vi "Configure Frequency Voltage Range.vi"(6 "Display (0: Primary Display)":i32(ring) items=["Primary Display", "Secondary Display"], 8 "error in (no error)":errorcluster, 9 "Manual Range (10)":dbl=10.0, 10 "Enable Frequency Voltage Auto Range (T:Enable)":bool=TRUE, 11 "VISA resource name":refnum<visa-resource-name>) -> (0 "error out":errorcluster, 3 "VISA resource name out":refnum<visa-resource-name>)   [LabVIEW 2020, in "Agilent 34405.lvlib"]
doc: "Configures the voltage range for Frequency measurement on the instrument.\n\n<B>Notes:</B>\n(1) This VI is only valid if the measurement function is set to Frequency."
uses:
  <instrlib>/Agilent 34405/Agilent 34405.lvlib
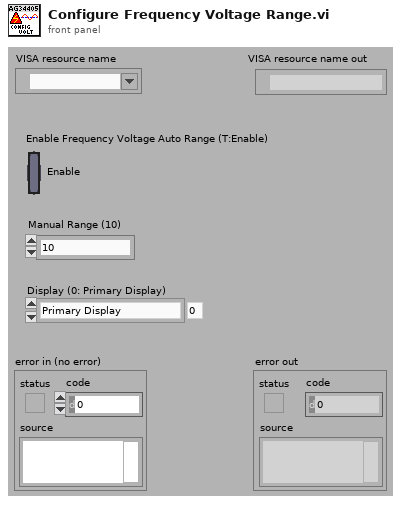
[diagram p1: front panel]
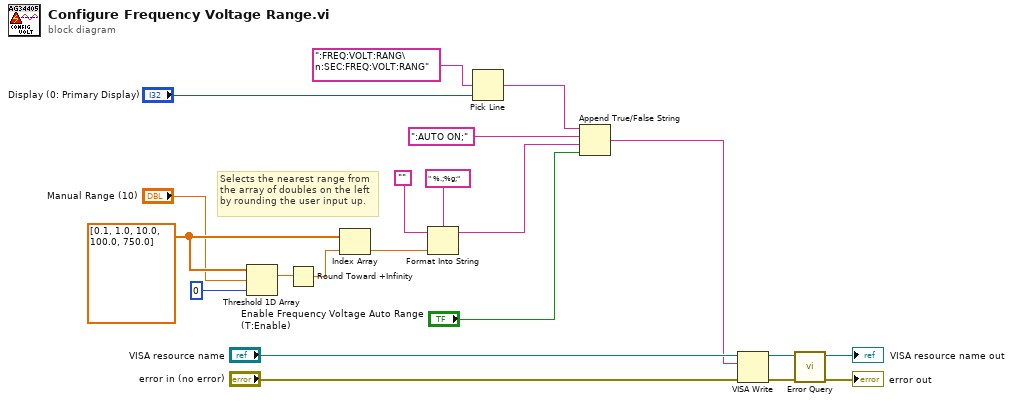
[diagram p0: block diagram]
diagram:
  w13 = dbl[] [0.1, 1.0, 10.0, 100.0, 750.0]
  # "Selects the nearest range from the array of doubles on the left by rounding the user input up."
  n1 = Threshold 1D Array(1:0 ("start index (0)"), 2:"Manual Range (10)", 3:w13) -> (0:w14:dbl)
  n2 = Round Toward +Infinity ("Round To +Infinity")(x=w14) -> (ceil(x): smallest int >= x=w12:dbl)
  n3 = Index Array(array=w13, index=w12) -> (element=w11:dbl)
  n4 = Format Into String(format string=" %.;%g;", initial string="" ("Empty String Constant"), w11) -> (resulting string=w6:string)  [unwired: 1 in, 1 out]
  n5 = Pick Line(multi-line string=":FREQ:VOLT:RANG\n:SEC:FREQ:VOLT:RANG" ("string"), line index="Display (0: Primary Display)") -> (output string=w1:string)  [unwired: 1 in]
  n6 = Append True/False String(1:"Enable Frequency Voltage Auto Range (T:Enable)", 2:w6, 3:":AUTO ON;" ("string"), 4:w1) -> (0:w5:string)
  n7 = VISA Write(VISA resource name="VISA resource name", write buffer=w5, error in (no error)="error in (no error)") -> (VISA resource name out=w21:refnum<visa-resource-name>, error out=w20:errorcluster)  [unwired: 1 out]
  n8 = call <instrlib>:"Error Query.vi"("error in (no error)"=w20, "VISA resource name"=w21) -> ("error out"=→"error out":errorcluster, "VISA resource name out"=→"VISA resource name out":refnum<visa-resource-name>)  [unwired: 8 out]
